vi "Read T0.vi"(8 "error in (no error)":errorcluster, 11 "PmuBase in":refnum<class "PmuBase.lvclass">) -> (0 "error out":errorcluster, 2 "T0":ext, 3 "PmuBase out":refnum<class "PmuBase.lvclass">)   [LabVIEW 2014]
uses:
  PmuBase.lvclass
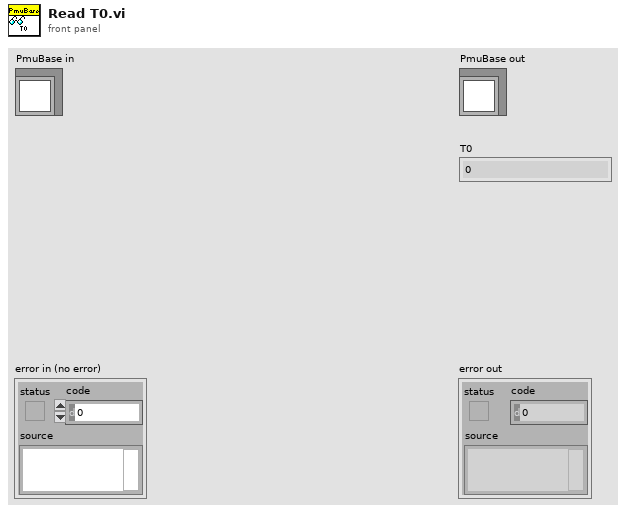
[diagram p1: front panel]
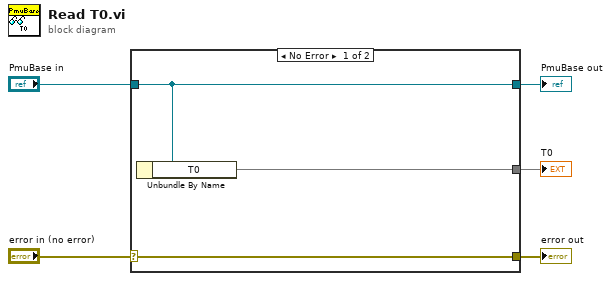
[diagram p0: block diagram]
diagram:
  n1 = case shown="No Error" "error in (no error)" {
    selector: "error in (no error)" -> [w8 w9]
    tunnel: [w8 w9] -> w4
    tunnel: [w7 w10] -> w2
    tunnel: "PmuBase in" -> [w7 w10]
    tunnel: [w6 _] -> w1
    frame No Error {
      n2 = Unbundle By Name(w7) -> ("T0"=w6)
    }
    frame Error {
    }
  }
  "error out" <- w4
  "PmuBase out" <- w2
  "T0" <- w1
